vi "Read_OTParamters.vi"() -> ()   [LabVIEW 2016]
uses:
  <vilib>/NI/Current Value Table/DataTypes/U16_Read.vi
  <vilib>/NI/Current Value Table/Type to Enum.vi
  <vilib>/NI/Current Value Table/DataTypes/U16_Type To Enum.vi
  <vilib>/Utility/file.llb/Read Delimited Spreadsheet (string).vi
  <vilib>/NI/Current Value Table/FGVs/CVT Globals.vi
  <vilib>/NI/Current Value Table/FGVs/Tag Memory.vi
  <vilib>/NI/Current Value Table/Memory Block.vi
  <vilib>/NI/Current Value Table/DataTypes/U16_Memory Block.vi
  <vilib>/NI/Current Value Table/Current Value Table.lvlib
panel:
  in  "Cancel Button":bool
  out "?":cluster{u16}[](array[cluster])
  out "?":cluster{u16}[](array[cluster])
  out "?":cluster{u16}[](array[cluster])
  out "?":cluster{u16}[](array[cluster])
  out "?":cluster{u16}[](array[cluster])
  out "?":cluster{u16}[](array[cluster])
  out "?":cluster{u16}[](array[cluster])
  out "?":cluster{u16}[](array[cluster])
  # "O.T Parameters"
  # "Bar"
  # "O2 Gas Pressure"
  # "Bar"
  # "N2 Gas Pressure 1"
  # "ft/m"
  # "Velocity"
  # "Bar"
  # "N2 Gas Pressure 2"
  # "Degree C"
  # "Room Temperature"
  # "%"
  # "Relative Humidity"
  # "Spare AI 01"
  # "Spare AI 02"
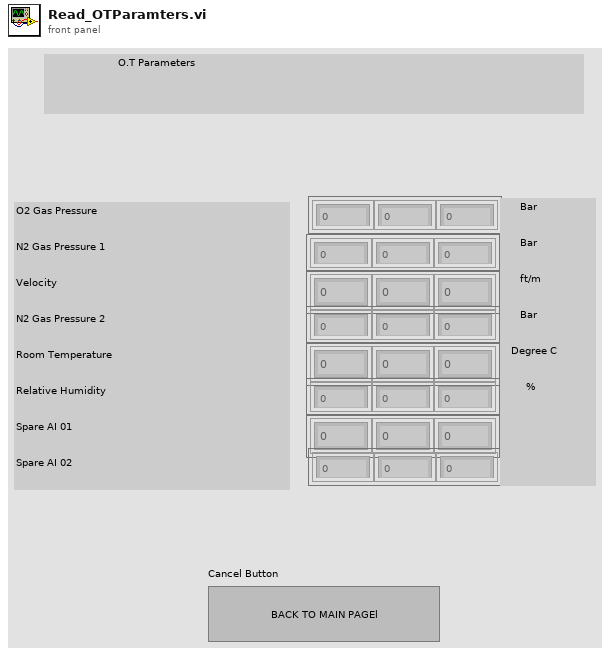
[diagram p1: front panel]
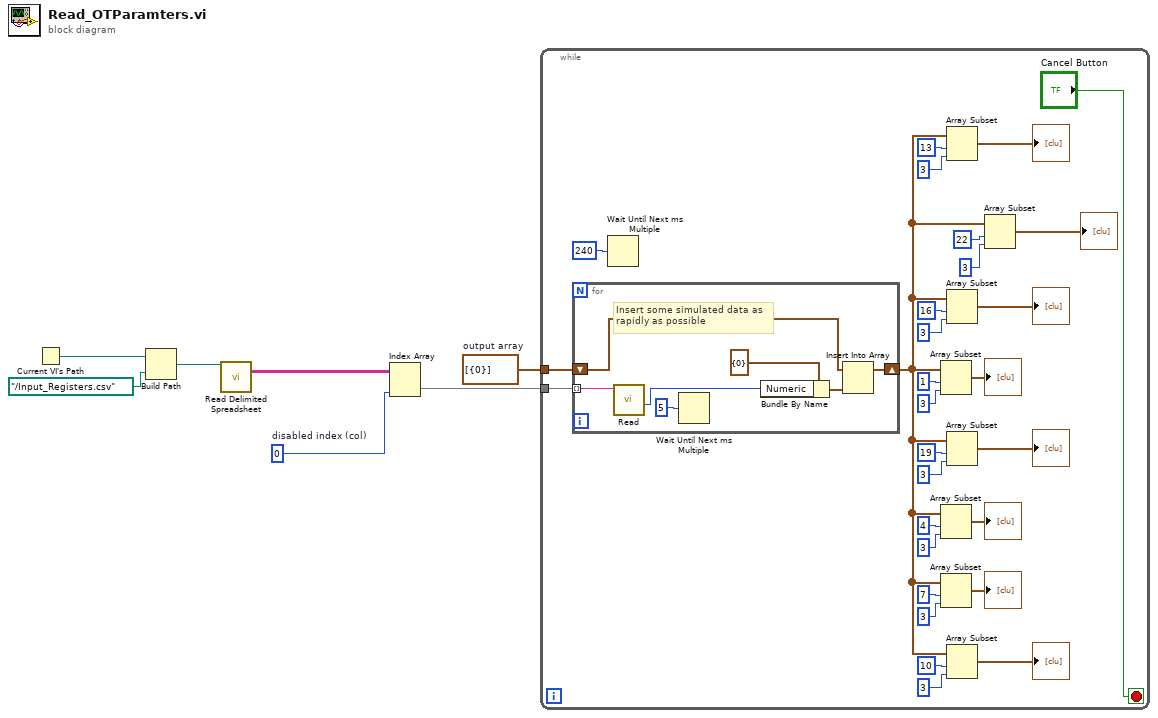
[diagram p0: block diagram]
diagram:
  w5 = cluster{"Numeric":u16}[] [{"Numeric"=0}]  # output array
  w7 = 0  # disabled index (col)
  n1 = Current VI's Path() -> (path=w3:path)
  n2 = Build Path(base path=w3, name or relative path=path "../Input_Registers.csv") -> (appended path=w1:path)
  n3 = call-poly <vilib>:"Read Delimited Spreadsheet.vi"("file path (dialog if empty)"=w1) -> ("all rows"=w6:string[][])  [unwired: 9 in, 5 out]
  n4 = Index Array "Index Array"(array=w6, index (col)=w7) -> (element=w4:string[])  [unwired: 1 in]
  n5 = while {
    tunnel: w5 -> [w36]
    tunnel: w4 -> [w35]
    stop <- "Cancel Button" stop-if-true
    n6 = for {
      shift-right: [w40] -> w12
      shift-left: w36 -> [w41]
      tunnel: w35 -> [w39] mode=indexing
      # "Insert some simulated data as\nrapidly as possible"
      n7 = call-poly <vilib>:"Read.vi"("Tag Name"=w39) -> ("Value"=w38:u16)  [unwired: 9 in, 1 out]
      n8 = Wait Until Next ms Multiple(millisecond multiple=u32 5 ("millisecond timer value")) -> ()  [unwired: 1 out]
      n9 = Bundle By Name(cluster=cluster{"Numeric":u16} {"Numeric"=0} ("Cluster"), "Numeric"=w38) -> (w42:cluster{"Numeric":u16})
      n10 = Insert Into Array(array=w41, new element=w42) -> (w40:cluster{"Numeric":u16}[])  [unwired: 1 in]
    }
    n11 = Wait Until Next ms Multiple(millisecond multiple=u32 240) -> ()  [unwired: 1 out]
    n12 = Array Subset(array=w12, index=1, length=3) -> (→"?":cluster{"Numeric":u16}[])
    n13 = Array Subset(array=w12, index=4, length=3) -> (→"?":cluster{"Numeric":u16}[])
    n14 = Array Subset(array=w12, index=7, length=3) -> (→"?":cluster{"Numeric":u16}[])
    n15 = Array Subset(array=w12, index=13, length=3) -> (→"?":cluster{"Numeric":u16}[])
    n16 = Array Subset(array=w12, index=16, length=3) -> (→"?":cluster{"Numeric":u16}[])
    n17 = Array Subset(array=w12, index=19, length=3) -> (→"?":cluster{"Numeric":u16}[])
    n18 = Array Subset(array=w12, index=10, length=3) -> (→"?":cluster{"Numeric":u16}[])
    n19 = Array Subset "Array Subset"(array=w12, index=22, length=3) -> (→"?":cluster{"Numeric":u16}[])
  }
